vi "skip.vi"(7 "custom report message (\"\")":string, 8 "error in (no error)":errorcluster, 10 "skipMessage":string, 11 "TestCase in":refnum<class "TestCase.lvclass">) -> (0 "error out":errorcluster, 3 "TestCase out":refnum<class "TestCase.lvclass">)   [LabVIEW 2013, in "TestCase.lvclass"]
doc: "If called within a running test, it will signal to the Test Runner that the test was skipped. If called before a test is actually run, it will causes the test to be skipped (and not actually run). \n\nskipMessage can be used to document a reason the test was skipped during test execution."
uses:
  TestCase.lvclass
  TestCase.lvclass/TestCase.ctl
panel:
  # "JKI VI Tester for LabVIEW\nhttp://jkisoft.com/vi-tester\nCopyright (C) 2007-2009, JKI <info@jkisoft.com>\nALL RIGHTS RESERVED"
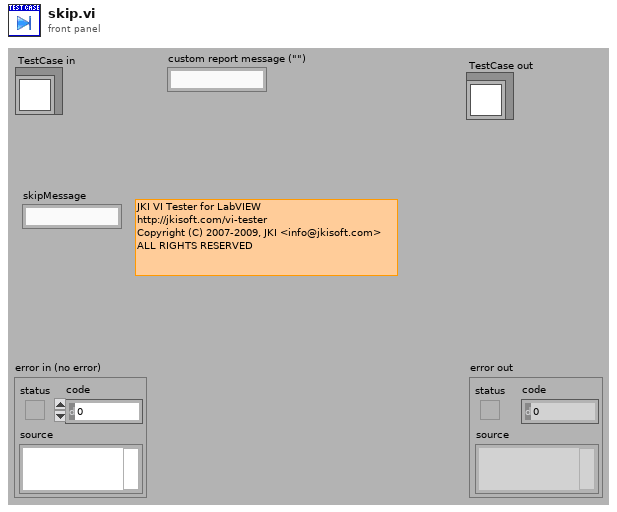
[diagram p1: front panel]
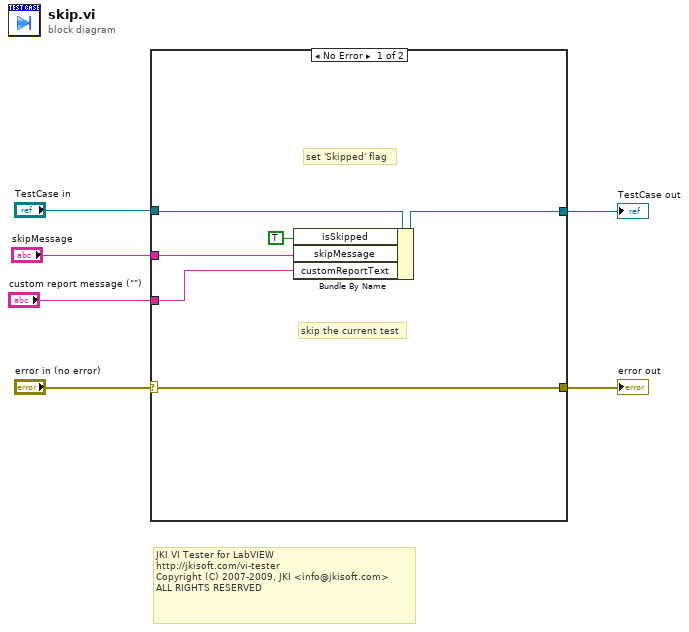
[diagram p0: block diagram]
diagram:
  # "JKI VI Tester for LabVIEW\nhttp://jkisoft.com/vi-tester\nCopyright (C) 2007-2009, JKI <info@jkisoft.com>\nALL RIGHTS RESERVED"
  n1 = case shown="No Error" "error in (no error)" {
    selector: "error in (no error)" -> [w12 w14]
    tunnel: [w12 w14] -> w5
    tunnel: [w9 w13] -> w3
    tunnel: "TestCase in" -> [w10 w13]
    tunnel: "skipMessage" -> [w8 _]
    tunnel: "custom report message (\"\")" -> [w7 _]
    frame No Error {
      # "set 'Skipped' flag"
      # "skip the current test"
      n2 = Bundle By Name(cluster=w10, "isSkipped"=TRUE, "skipMessage"=w8, "customReportText"=w7) -> (w9:refnum<class "TestCase.lvclass">)
    }
    frame Error {
    }
  }
  "error out" <- w5
  "TestCase out" <- w3
